vi "Build_URL.vi"(8 "error in (no error)":errorcluster, 11 "Request in":refnum<class "Request.lvclass">) -> (0 "error out":errorcluster, 3 "Request out":refnum<class "Request.lvclass">)   [LabVIEW 2016, in "Request.lvclass"]
uses:
  Request.lvclass
  <vilib>/Utility/error.llb/whitespace.ctl
  Request.lvclass/Request.ctl
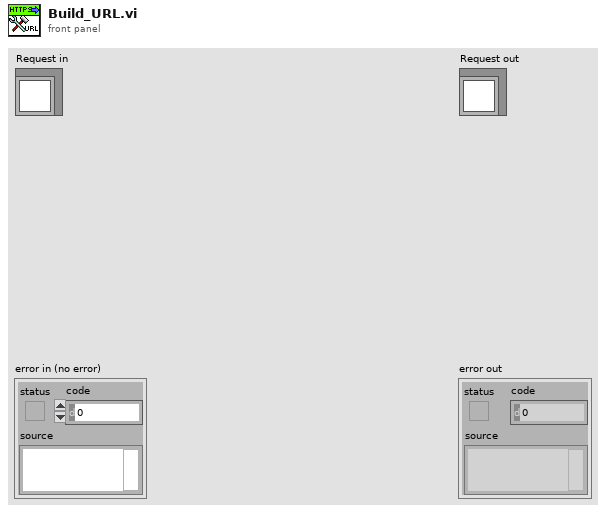
[diagram p1: front panel]
types:
  T1 = typedef "whitespace.ctl" = u16
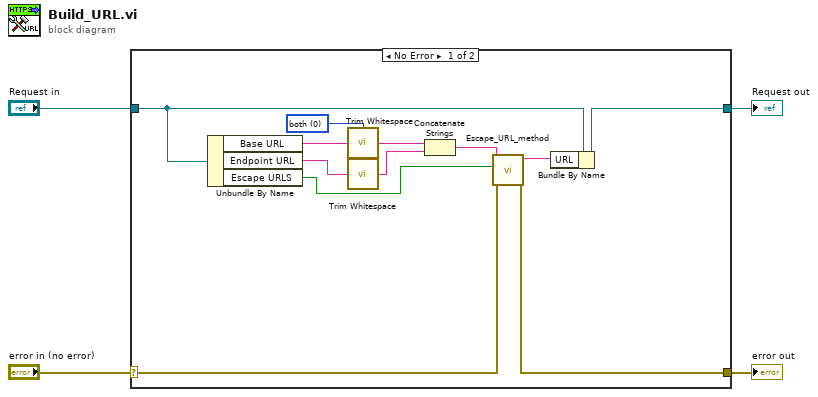
[diagram p0: block diagram]
diagram:
  n1 = case shown="No Error" "error in (no error)" {
    selector: "error in (no error)" -> [w10 w18]
    tunnel: [w9 w18] -> w3
    tunnel: [w7 w17] -> w1
    tunnel: "Request in" -> [w8 w17]
    frame No Error {
      w12 = T1 0 items=["both", "start of string", "end of string"] ("location (both)")
      n2 = Unbundle By Name(w8) -> ("Base URL"=w16:string, "Endpoint URL"=w15:string, "Escape URLS"=w5:bool)
      n3 = call <vilib>:"Trim Whitespace.vi"("string"=w16, "location (both)"=w12) -> ("trimmed string"=w14:string)
      n4 = call <vilib>:"Trim Whitespace.vi"("string"=w15, "location (both)"=w12) -> ("trimmed string"=w13:string)
      n5 = Concatenate Strings(w14, w13) -> (w11:string)
      n6 = call "Escape_URL_method.vi"("error in (no error)"=w10, "Escape URLs?"=w5, "URL In"=w11) -> ("error out"=w9:errorcluster, "URL Out"=w6:string)  [unwired: 7 in]
      n7 = Bundle By Name(cluster=w8, "URL"=w6) -> (w7:refnum<class "Request.lvclass">)
    }
    frame Error {
    }
  }
  "error out" <- w3
  "Request out" <- w1
